vi "Instrument Level Controls.vi"(8 "error in (no error)":errorcluster, 11 "MIDI Controls in":variant) -> (0 "error out":errorcluster, 2 "Instrument Level Controls out":variant)   [LabVIEW 2014, in "mySynthesizer.lvlib" / "Instrument Level Controls.lvlib"]
uses:
  Instrument Level Controls.lvlib
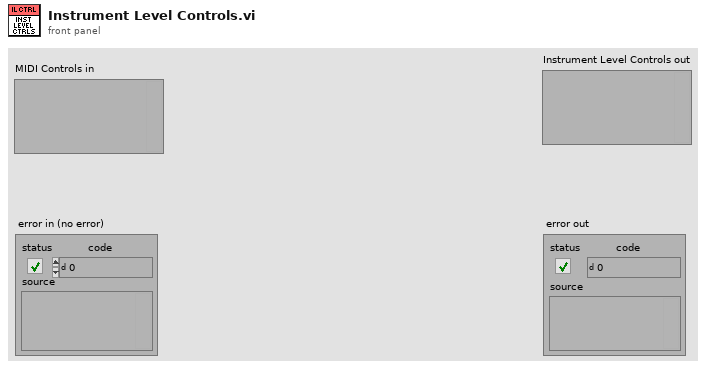
[diagram p1: front panel]
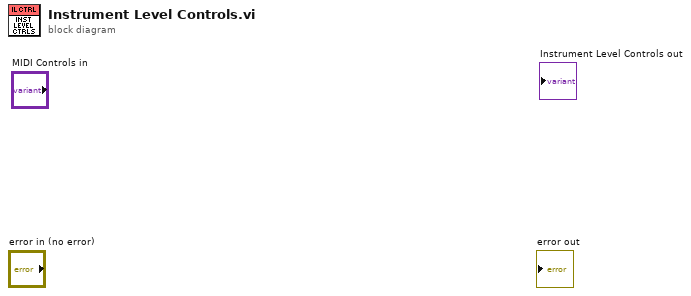
[diagram p0: block diagram]
diagram:
